vi "Show Front Panel (poly).vi"   [LabVIEW 2024, in "Module.lvclass"]
uses:
  Module.lvclass
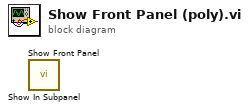
[diagram p0: block diagram]
diagram:
  n1 = call "Show In Subpanel.vi"() -> ()  [unwired: 10 in, 2 out]
  n2 = call "Show Front Panel.vi"() -> ()  [unwired: 10 in, 2 out]
